vi "Pump Status Pump Module.vi"(8 "error in (no error)":errorcluster, 11 "?":T1={"State"=enum."Idle", "Start Time"=timestamp(0 s since 1904-01-01), "Configuration"={"Cycle Period"=0.0, "Manual Entry"=0.0, "Output Device"=enum."VICI M6", "Ismatech"={"VISA resource name"="", "Simulated?"=FALSE, "Pump Number"=1.0, "Reverse?"=FALSE}, "Ismatech 3 Channel Settings"={"VISA resource name"="", "Pump Number"=1, "Channel Number"=0, "Simulated?"=TRUE, "Reverse?"=FALSE}, "Masterflex"={"VISA resource name"="", "Simulated?"=FALSE, "Pump Number"=1.0, "Reverse?"=FALSE}, "VICI Settings"={"VISA resource name"="", "Pump ID"="", "Pump Head Vol"=0.0, "Reverse?"=FALSE, "Simulated?"=FALSE}, "Tacmina Settings"={"Analog DAQ Task"="", "Digital DAQ Task"=""}, "KNF SIMDOS Settings"={"VISA resource name"="", "Simulated?"=TRUE}, "ASIA Pump C"={"ASIA Pump #"=0, "channel"=0, "Simulated"=FALSE}, "FLOM Settings"={"VISA resource name"="", "Simulated?"=TRUE, "Pump Number"=0.0}, "SSI PR/LD Settings"={"VISA resource name"="", "Simulated?"=FALSE}, "SSI P40 Settings"={"VISA resource name"="", "Simulated?"=FALSE}, "Masterflex 75211 Settings"={"Analog DAQ Task"="", "Digital DAQ Task"=""}, "Pump Calibration File"=path "", "Calibration Slope"=0.0, "Calibration Y Intercept"=0.0, "Pump Cal Enum"=0, "Reset Totalizer"=FALSE}, "Current Time"=timestamp(0 s since 1904-01-01), "First Iteration"=FALSE, "Data"={"Pump Speed"=0.0, "Pump Pressure"=0.0, "Pump Flow"=0.0, "Totalized"=0.0}, "Process Name"="", "Pump On?"=enum."Off", "Output Error"=FALSE, "Log Started"=FALSE, "Overpressure Alarming"=FALSE} {"Configuration"."Ismatech 3 Channel Settings"."Channel Number" min=0 max=3; "Configuration"."Ismatech 3 Channel Settings"."Pump Number" min=1; "Configuration"."ASIA Pump C"."channel" min=0 max=1 step=1; "Configuration"."Masterflex"."Pump Number" min=1.0 max=20.0 step=1.0; "Configuration"."Ismatech"."Pump Number" min=1.0 max=20.0 step=1.0}) -> (0 "error out":errorcluster, 3 "State out":T1={"State"=enum."Idle", "Start Time"=timestamp(0 s since 1904-01-01), "Configuration"={"Cycle Period"=0.0, "Manual Entry"=0.0, "Output Device"=enum."Ismatec ISM 831C", "Ismatech"={"VISA resource name"="", "Simulated?"=FALSE, "Pump Number"=1.0, "Reverse?"=FALSE}, "Ismatech 3 Channel Settings"={"VISA resource name"="", "Pump Number"=1, "Channel Number"=0, "Simulated?"=TRUE, "Reverse?"=FALSE}, "Masterflex"={"VISA resource name"="", "Simulated?"=FALSE, "Pump Number"=1.0, "Reverse?"=FALSE}, "VICI Settings"={"VISA resource name"="", "Pump ID"="", "Pump Head Vol"=0.0, "Reverse?"=FALSE, "Simulated?"=FALSE}, "Tacmina Settings"={"Analog DAQ Task"="", "Digital DAQ Task"=""}, "KNF SIMDOS Settings"={"VISA resource name"="", "Simulated?"=TRUE}, "ASIA Pump C"={"ASIA Pump #"=0, "channel"=0, "Simulated"=FALSE}, "FLOM Settings"={"VISA resource name"="", "Simulated?"=TRUE, "Pump Number"=0.0}, "SSI PR/LD Settings"={"VISA resource name"="", "Simulated?"=FALSE}, "SSI P40 Settings"={"VISA resource name"="", "Simulated?"=FALSE}, "Masterflex 75211 Settings"={"Analog DAQ Task"="", "Digital DAQ Task"=""}, "Pump Calibration File"=path "", "Calibration Slope"=0.0, "Calibration Y Intercept"=0.0, "Pump Cal Enum"=0, "Reset Totalizer"=FALSE}, "Current Time"=timestamp(0 s since 1904-01-01), "First Iteration"=FALSE, "Data"={"Pump Speed"=0.0, "Pump Pressure"=0.0, "Pump Flow"=0.0, "Totalized"=0.0}, "Process Name"="", "Pump On?"=enum."Off", "Output Error"=FALSE, "Log Started"=FALSE, "Overpressure Alarming"=FALSE} {"Configuration"."Ismatech 3 Channel Settings"."Channel Number" min=0 max=3; "Configuration"."Ismatech 3 Channel Settings"."Pump Number" min=1; "Configuration"."ASIA Pump C"."channel" min=0 max=1 step=1; "Configuration"."Masterflex"."Pump Number" min=1.0 max=20.0 step=1.0; "Configuration"."Ismatech"."Pump Number" min=1.0 max=20.0 step=1.0})   [LabVIEW 2018, in "Pump Module.lvlib"]
uses:
  Pump Module.lvlib
  Measure Instrument/State Cluster.ctl
  Measure Instrument/State Enum.ctl
  Pump Module Settings Cluster.ctl
  Measure Instrument/PID 2 Output Enum.ctl
  Ismatec ISM 831C/Controls/Ismatech ISM831C Settings Cluster.ctl
  Ismatec 78001/Ismatec 4083.ctl
  Masterflex 7550-30/Controls/Settings Cluster.ctl
  VICI M50 Party Mode/Settings Cluster.ctl
  Tacmina QI/Tacmina QI DAQ Setting.ctl
  KNF Pump/Settings Cluster plus SIMDOS.ctl
  ASIA Pump/Pump Settings.ctl
  FLOM Pump/Settings Cluster.ctl
  SSI PR Class/SSI PR or LD Settings Cluster.ctl
  Masterflex 75211/Masterflex 75211 DAQ Setting.ctl
  Tag VIs/Tag FGV Operation Enum.ctl
  Ismatec ISM 831C/Ismatec ISM 831C.lvlib
  Masterflex 7550-30/Masterflex 7550-30.lvlib
  Shared Variables/Dynamic Shared Variables.lvlib
  Measure Instrument/Pump Module Engine.lvlib
  Tacmina QI/Tacmina QI.lvlib
  KNF Pump/KNF SIMDOS.lvlib
  VICI M50 Party Mode/VICI M6 M50 Party Mode.lvlib
  FLOM Pump/FLOM Pump.lvlib
  ASIA Pump.lvlib
  SSI PR Class/SSI PR or LD Pump.lvlib
  Masterflex 75211/Masterflex 75211.lvlib
  SSI PR Class/SSI P40 Pump.lvlib
  Ismatec 78001/Ismatec 4308.lvlib
panel:
  # "Output Instruments"
  # "Output Instruments"
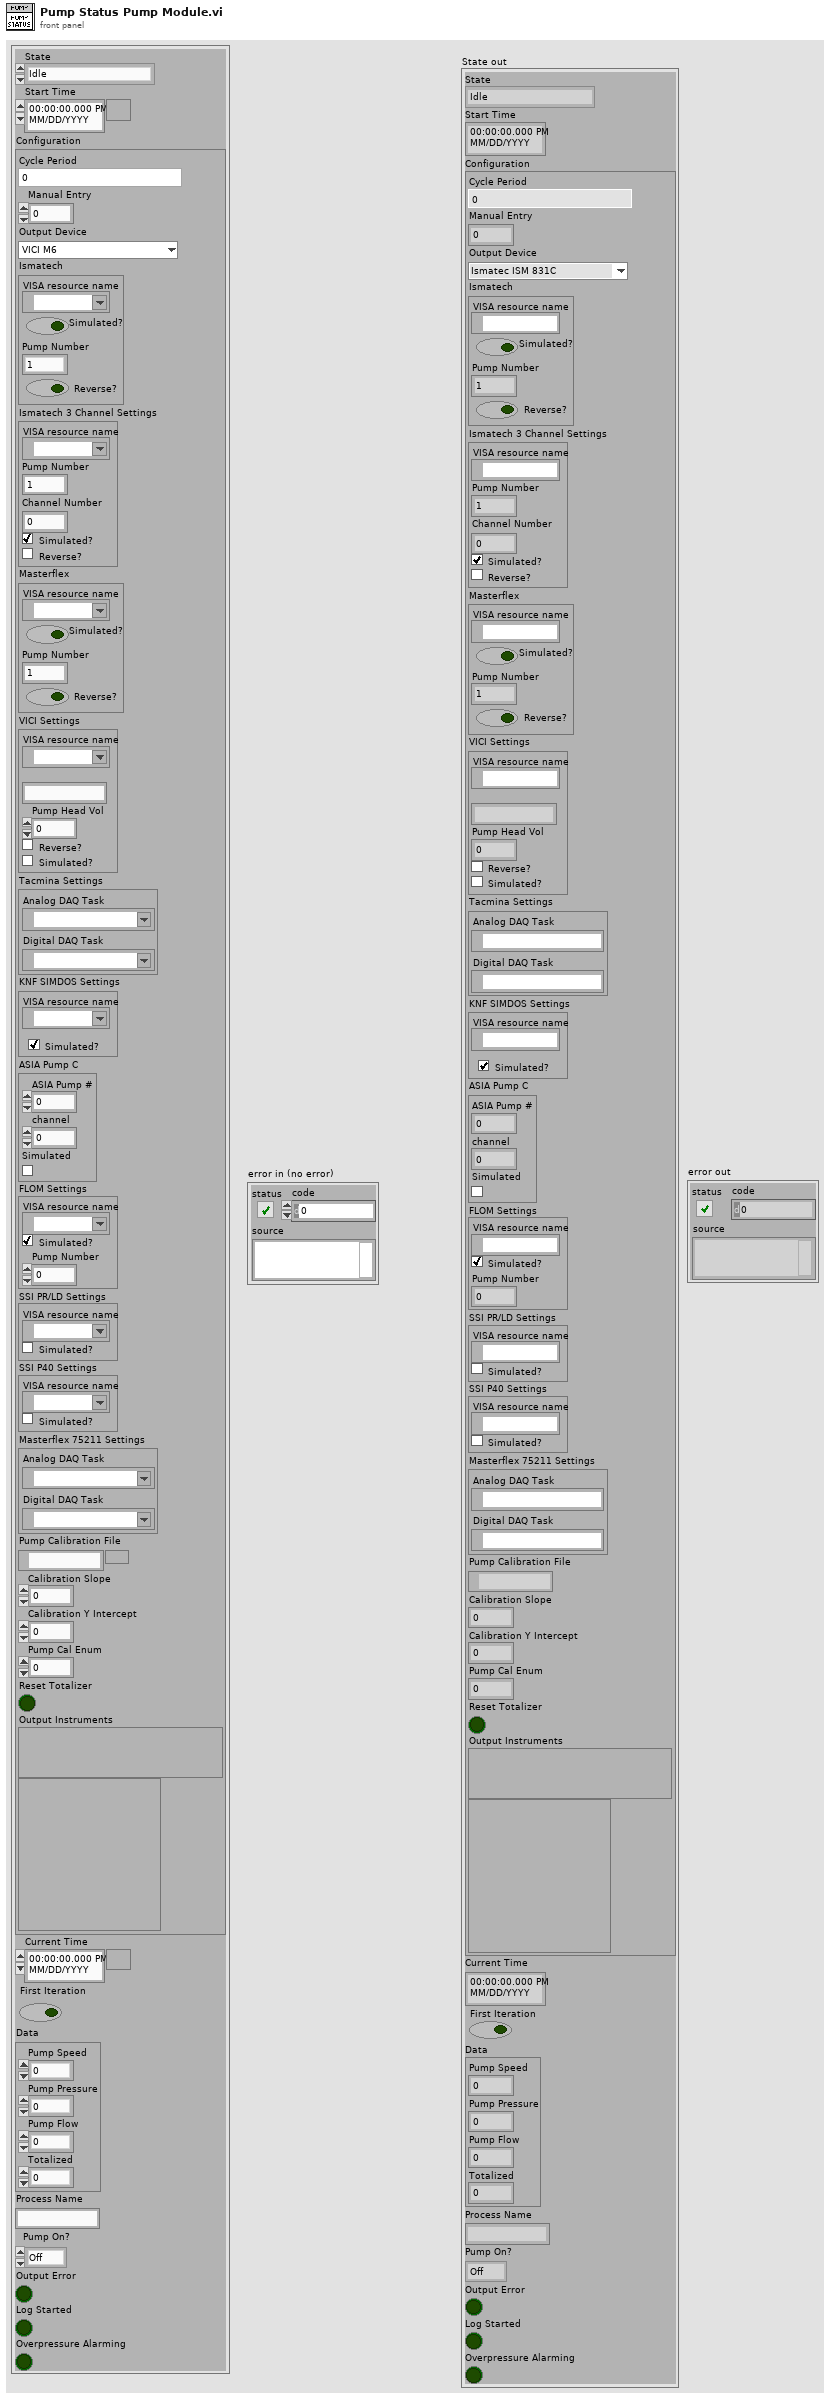
[diagram p1: front panel]
types:
  T1 = typedef "Pump Module.lvlib/Pump Module Engine.lvlib/State Cluster.ctl" = cluster{"State":T2, "Start Time":timestamp, "Configuration":T3, "Current Time":timestamp, "First Iteration":bool, "Data":cluster{"Pump Speed":dbl, "Pump Pressure":dbl, "Pump Flow":dbl, "Totalized":dbl}, "Process Name":string, "Pump On?":enum16{"Off", "On", "Not Initialized"}, "Output Error":bool, "Log Started":bool, "Overpressure Alarming":bool}
  T2 = typedef "Pump Module.lvlib/Pump Module Engine.lvlib/State Enum.ctl" = enum16{"Measuring", "Idle", "Paused"}
  T3 = typedef "Pump Module.lvlib/Pump Module Settings Cluster.ctl" = cluster{"Cycle Period":dbl, "Manual Entry":dbl, "Output Device":T4, "Ismatech":T5, "Ismatech 3 Channel Settings":T6, "Masterflex":T7, "VICI Settings":T8, "Tacmina Settings":T9, "KNF SIMDOS Settings":T10, "ASIA Pump C":T11, "FLOM Settings":T12, "SSI PR/LD Settings":T13, "SSI P40 Settings":T13, "Masterflex 75211 Settings":T14, "Pump Calibration File":path, "Calibration Slope":dbl, "Calibration Y Intercept":dbl, "Pump Cal Enum":u16, "Reset Totalizer":bool}
  T4 = typedef "PID 2 Output Enum.ctl" = enum16{"Default", "Ismatec ISM 4308", "Ismatec ISM 831C", "Masterflex 7550-30", "VICI M6", "VICI M50", "Tacmina QI", "KNF SIMDOS", "ASIA Type C", "FLOM UI-22-11", "SSI PR/LD", "SSI P40", "Masterflex 75211-70"}
  T5 = typedef "Ismatec ISM 831C.lvlib/Ismatech ISM831C Settings Cluster.ctl" = cluster{"VISA resource name":refnum<visa-resource-name>, "Simulated?":bool, "Pump Number":dbl, "Reverse?":bool}
  T6 = typedef "Ismatec 4308.lvlib/Ismatec 4083.ctl" = cluster{"VISA resource name":refnum<visa-resource-name>, "Pump Number":i16, "Channel Number":i16, "Simulated?":bool, "Reverse?":bool}
  T7 = typedef "Masterflex 7550-30.lvlib/Settings Cluster.ctl" = cluster{"VISA resource name":refnum<visa-resource-name>, "Simulated?":bool, "Pump Number":dbl, "Reverse?":bool}
  T8 = typedef "VICI M6 M50 Party Mode.lvlib/Settings Cluster.ctl" = cluster{"VISA resource name":refnum<visa-resource-name>, "Pump ID":string, "Pump Head Vol":dbl, "Reverse?":bool, "Simulated?":bool}
  T9 = typedef "Tacmina QI.lvlib/Tacmina QI DAQ Setting.ctl" = cluster{"Analog DAQ Task":refnum<k21>, "Digital DAQ Task":refnum<k21>}
  T10 = typedef "KNF SIMDOS.lvlib/Settings Cluster plus SIMDOS.ctl" = cluster{"VISA resource name":refnum<visa-resource-name>, "Simulated?":bool}
  T11 = typedef "ASIA Pump.lvlib/Pump Settings.ctl" = cluster{"ASIA Pump #":i32, "channel":i32, "Simulated":bool}
  T12 = typedef "FLOM Pump.lvlib/Settings Cluster.ctl" = cluster{"VISA resource name":refnum<visa-resource-name>, "Simulated?":bool, "Pump Number":dbl}
  T13 = typedef "SSI PR or LD Pump.lvlib/SSI PR or LD Settings Cluster.ctl" = cluster{"VISA resource name":refnum<visa-resource-name>, "Simulated?":bool}
  T14 = typedef "Masterflex 75211.lvlib/Masterflex 75211 DAQ Setting.ctl" = cluster{"Analog DAQ Task":refnum<k21>, "Digital DAQ Task":refnum<k21>}
  T15 = typedef "Tag FGV Operation Enum.ctl" = enum16{"Init", "Set Notification Queue", "Create Tag", "Commit", "Write Tag (Numeric)", "Write Tag (Boolean)", "Read All Tags", "Read One Tag", "Delete Tag Category", "Set Alarm Parameters (Numeric)", "Set Alarm Parameters (Boolean)", "Enable All Alarms", "Disable All Alarms", "Delete All Tags", "Read Alarms", "Ack Alarm", "Read Alarm Parameters (Numeric)", "Read Alarm Parameters (Boolean)"}
  T16 = typedef "Pump Module.lvlib/Pump Module Tag Names Cluster.ctl" = cluster{"Pump Speed":string, "Totalized g Tag":string, "Pump Flow":string, "Pump Pressure":string, "Output Device Tag":string, "Overpressure Tag":string, "Identifier Tag":string}
  T17 = cluster{"alarm URL":string, "set time":timestamp, "set user":string, "ack time":timestamp, "ack user":string, "clear time":timestamp, "clear user":string, "setpoint":dbl, "value":dbl, "priority":u32, "alarm area":string, "alarm description":string, "ack comment":string, "event?":bool, "Refnum":u64}[]
  T18 = typedef "Dynamic Shared Variables.lvlib/Alarm Cluster (UI).ctl" = cluster{"Color Box":u32, "Name":string, "Ack":bool}
  T19 = typedef "SSI P40 Pump.lvlib/SSI P40 Settings Cluster.ctl" = cluster{"VISA resource name":refnum<visa-resource-name>, "Simulated?":bool}
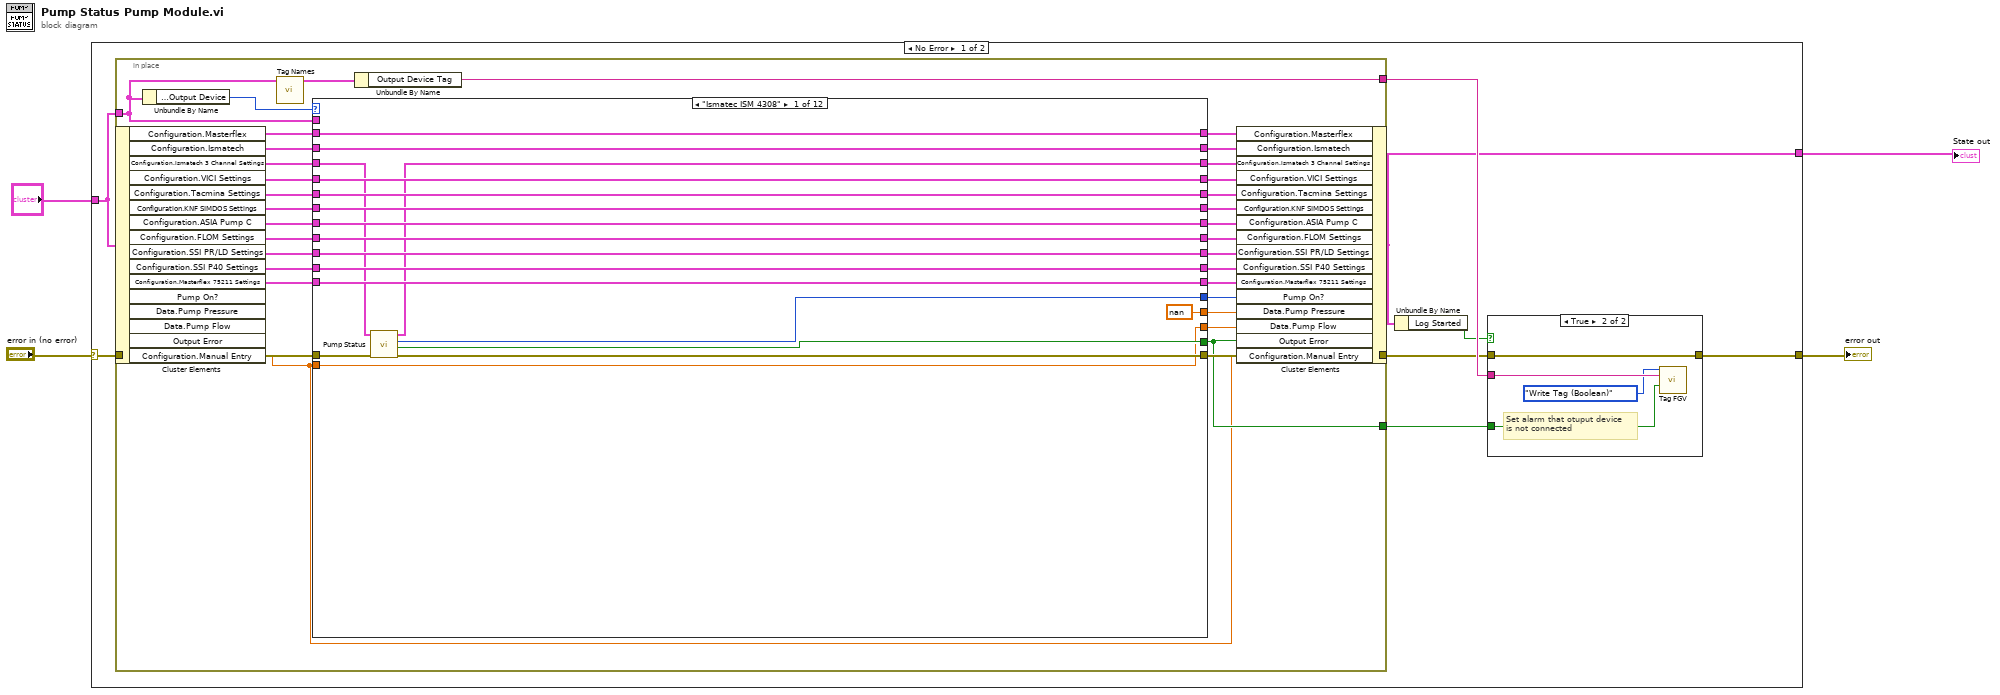
[diagram p0: block diagram]
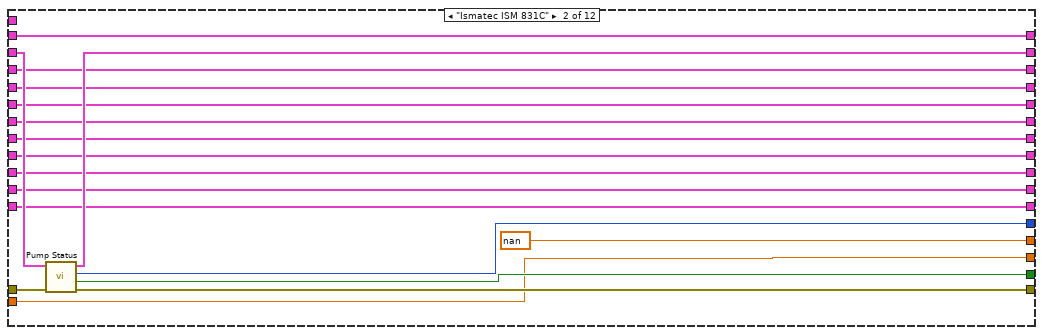
[diagram p2: hidden frame]
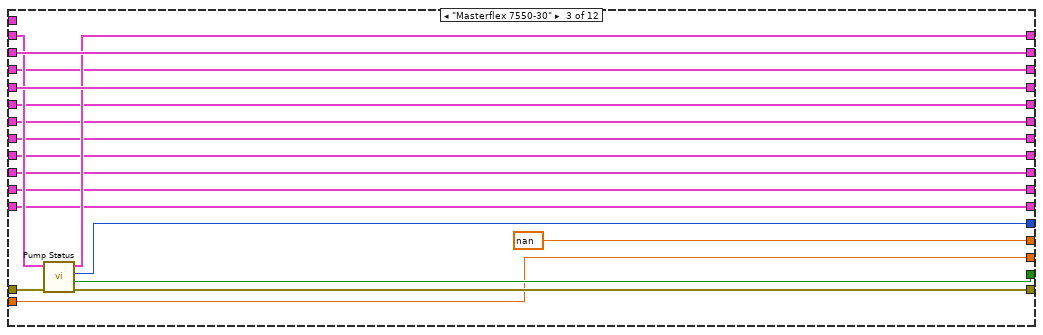
[diagram p3: hidden frame]
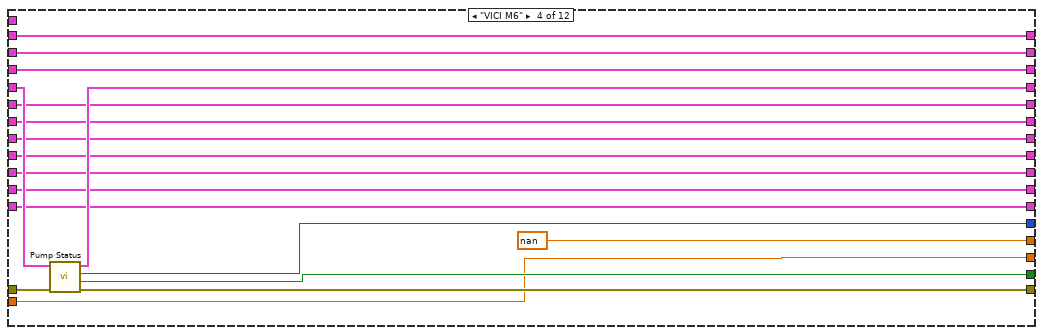
[diagram p4: hidden frame]
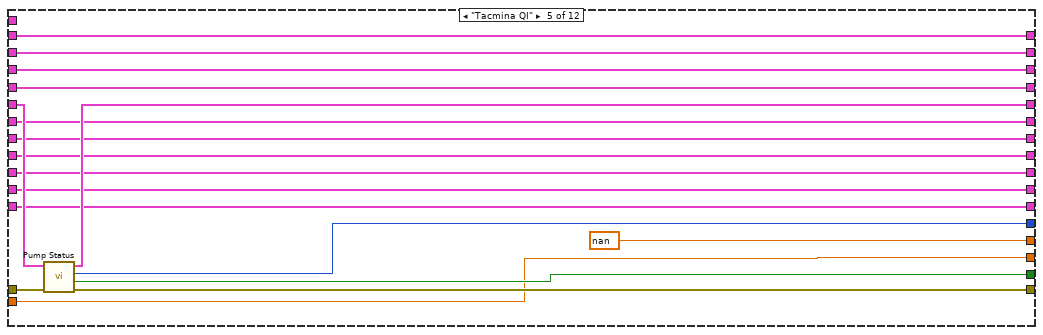
[diagram p5: hidden frame]
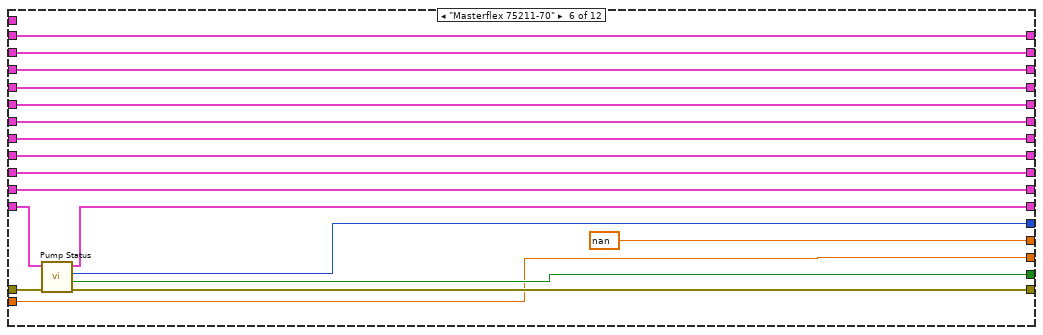
[diagram p6: hidden frame]
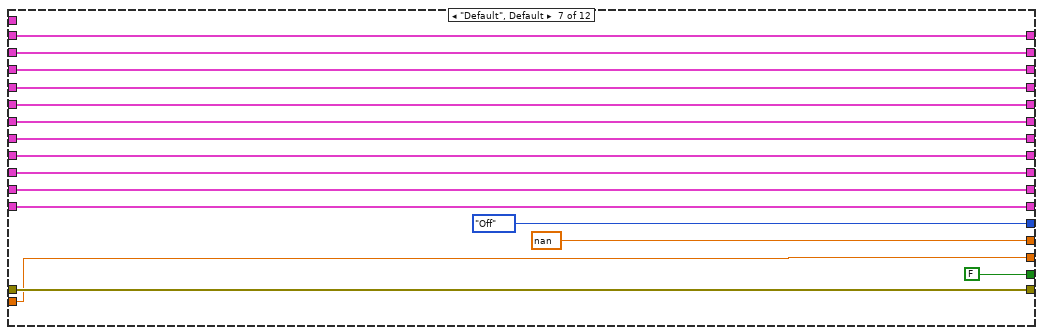
[diagram p7: hidden frame]
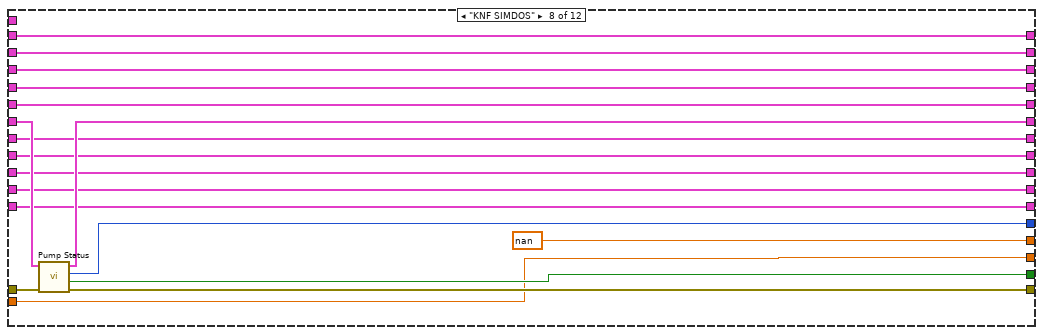
[diagram p8: hidden frame]
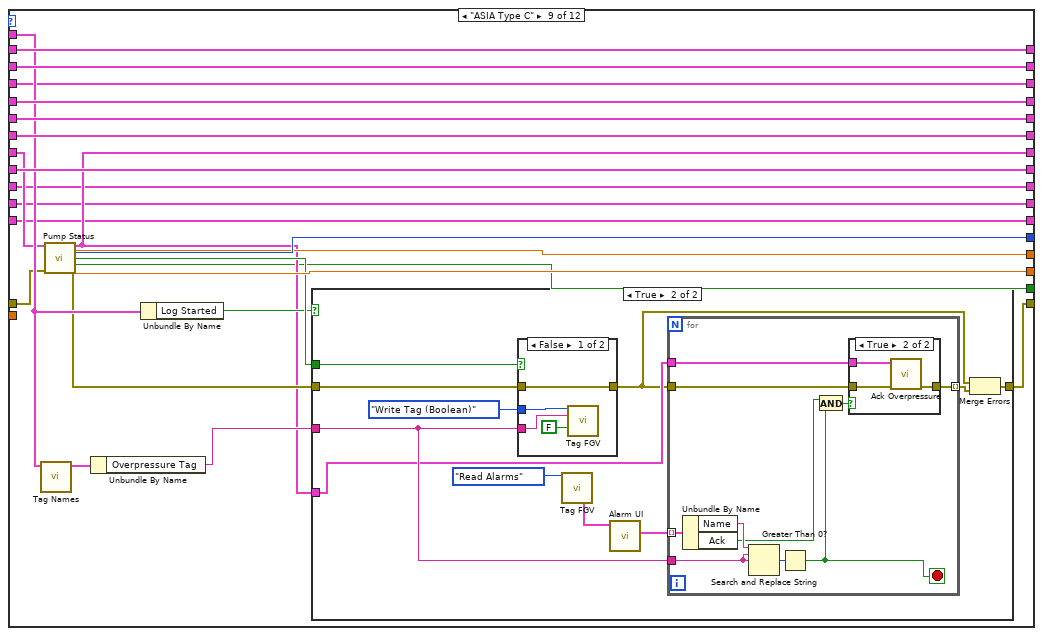
[diagram p9: hidden frame]
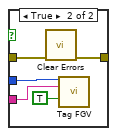
[diagram p12: hidden frame]
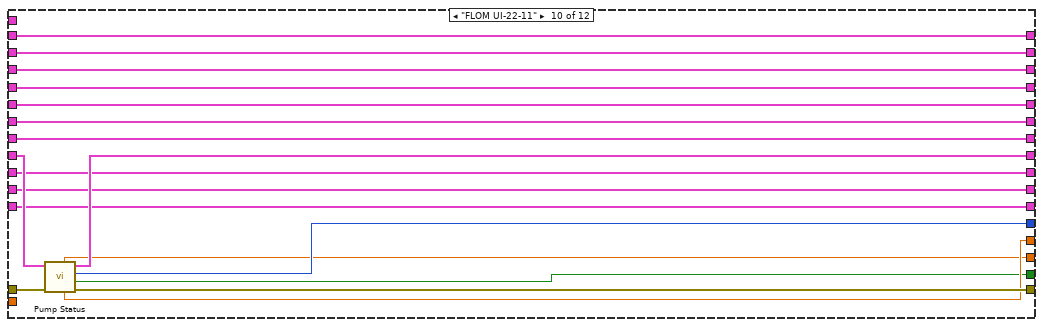
[diagram p13: hidden frame]
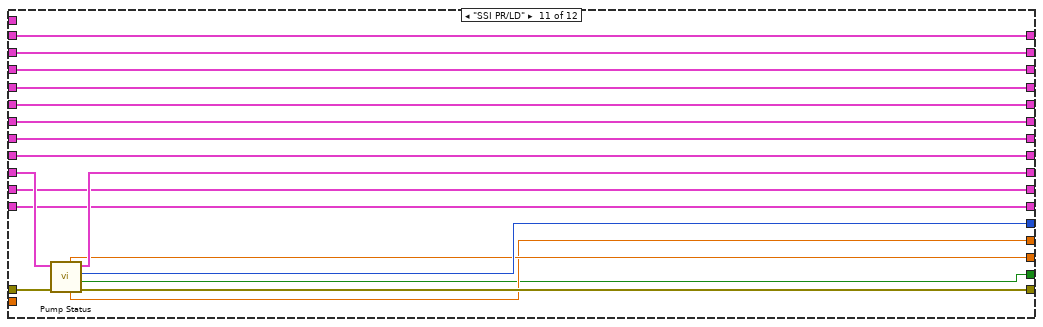
[diagram p14: hidden frame]
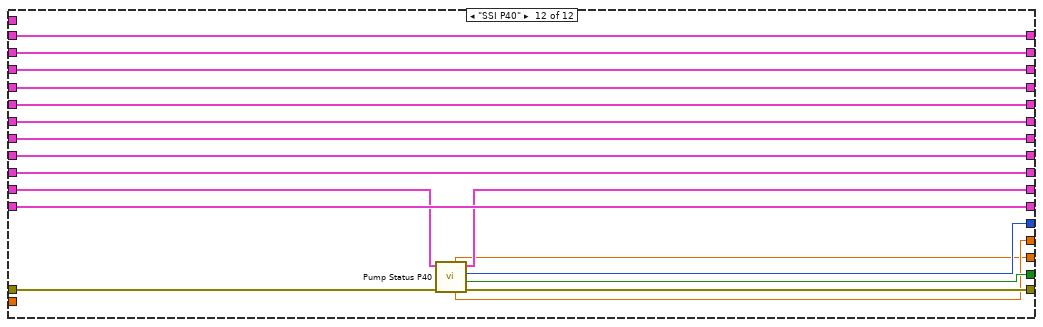
[diagram p15: hidden frame]
diagram:
  n1 = case shown="No Error" "error in (no error)" {
    selector: "error in (no error)" -> [w12 w307]
    tunnel: [w9 w307] -> w3
    tunnel: "?" -> [w6 w306]
    tunnel: [w5 w306] -> w1
    frame No Error {
      n2 = in-place {
        in-place-border: w12 -> [w45]
        in-place-border: [w44] -> w11
        in-place-border: [w43] -> w10
        in-place-border: w6 -> [w40]
        in-place-border: [w31] -> w7
        n3 = in-place-cluster #1(w6) -> ("Configuration.Masterflex"=w39:T7, "Configuration.Ismatech"=w38:T5, "Configuration.Ismatech 3 Channel Settings"=w16:T6, "Configuration.VICI Settings"=w37:T8, "Configuration.Tacmina Settings"=w36:T9, "Configuration.KNF SIMDOS Settings"=w35:T10, "Configuration.ASIA Pump C"=w34:T11, "Configuration.FLOM Settings"=w33:T12, "Configuration.SSI PR/LD Settings"=w32:T13, "Configuration.SSI P40 Settings"=w17:T13, "Configuration.Masterflex 75211 Settings"=w20:T14, "Configuration.Manual Entry"=w13:dbl)  [unwired: 4 out]
        n4 = Unbundle By Name(w40) -> ("Configuration.Output Device"=w41:T4)
        n5 = call "Tag Names.vi"("State In"=w40) -> ("Pump Module Tag Names"=w42:T16)  [unwired: 8 in, 2 out]
        n6 = case "Selected Device" shown="\"Ismatec ISM 4308\"" w41 {
          tunnel: w39 -> [w63 w81 w94 w116 w135 w153 w169 w187 w211 w264 w282 w292]
          tunnel: [w63 w81 w95 w116 w135 w153 w169 w187 w211 w264 w282 w292] -> w30
          tunnel: w38 -> [w62 w78 w99 w117 w134 w152 w168 w186 w210 w263 w281 w300]
          tunnel: [w50 w79 w96 w112 w130 w142 w166 w182 w194 w257 w272 w286] -> w43
          tunnel: w45 -> [w53 w80 w97 w113 w131 w145 w166 w183 w203 w258 w276 w291]
          tunnel: [w62 w77 w99 w117 w134 w152 w168 w186 w210 w263 w281 w300] -> w29
          tunnel: w37 -> [w61 w75 w98 w114 w133 w151 w167 w185 w209 w262 w280 w299]
          tunnel: [w61 w75 w98 w115 w133 w151 w167 w185 w209 w262 w280 w299] -> w28
          tunnel: w36 -> [w60 w76 w93 w111 w132 w141 w165 w184 w208 w261 w279 w298]
          tunnel: [w60 w76 w93 w111 w129 w141 w165 w184 w208 w261 w279 w298] -> w27
          tunnel: [w59 w74 w92 w110 w128 w150 w164 w181 w207 w260 w278 w297] -> w26
          tunnel: w35 -> [w59 w74 w92 w110 w128 w150 w164 w180 w207 w260 w278 w297]
          tunnel: [w48 w73 w90 w109 w127 w144 enum16{"Off", "On", "Not Initialized"}."Off" ("Pump On?") w179 w201 w254 w271 w288] -> w22
          tunnel: [w58 w72 w91 w108 w126 w149 w162 w178 w193 w259 w277 w296] -> w25
          tunnel: w34 -> [w58 w72 w91 w108 w126 w149 w162 w178 w202 w259 w277 w296]
          tunnel: [w57 w71 w89 w107 w125 w148 w161 w177 w206 w256 w275 w295] -> w24
          tunnel: w33 -> [w57 w71 w89 w107 w125 w148 w161 w177 w206 w255 w275 w295]
          tunnel: [w46 w64 w82 w100 w118 w136 w154 w170 w198 w252 w270 w284] -> w14
          tunnel: [nan ("Pressure") nan ("Pressure") nan ("Pressure") nan ("Pressure") nan ("Pressure") nan ("Pressure") nan ("Pressure") nan ("Pressure") w199 w253 w269 w285] -> w21
          tunnel: w40 -> [_ _ _ _ _ _ _ _ w204 _ _ _]
          tunnel: w32 -> [w56 w69 w87 w105 w123 w146 w159 w175 w192 w251 w274 w294]
          tunnel: [w56 w69 w87 w105 w123 w146 w159 w175 w192 w251 w273 w294] -> w23
          tunnel: [w49 w68 w86 w104 w122 w143 FALSE ("Connection Error") w174 w191 w250 w268 w287] -> w31
          tunnel: w20 -> [w55 w67 w85 w103 w121 w140 w157 w173 w190 w249 w267 w293]
          tunnel: [w55 w67 w85 w103 w121 w139 w157 w173 w190 w249 w267 w293] -> w19
          tunnel: [w54 w66 w84 w102 w120 w138 w156 w172 w189 w248 w266 w289] -> w18
          tunnel: w17 -> [w54 w66 w84 w102 w120 w138 w156 w172 w189 w248 w266 w290]
          tunnel: w16 -> [w52 w65 w83 w101 w119 w137 w155 w171 w188 w247 w265 w283]
          tunnel: [w51 w65 w83 w101 w119 w137 w155 w171 w188 w247 w265 w283] -> w15
          tunnel: w13 -> [w46 w64 w82 w100 w118 w136 w154 w170 _ _ _ _]
          frame "Ismatec ISM 4308" {
            n7 = call "Pump Status.vi"("error in (no error)"=w53, "Ismatech 3 Channel Settings In"=w52) -> ("error out"=w50:errorcluster, "Connection Error"=w49:bool, "Pump On?"=w48:enum16{"Off", "On", "Not Initialized"}, "Ismatech 3 Channel Settings Out"=w51:T6)  [unwired: 5 in, 1 out]
          }
          frame "Ismatec ISM 831C" {
            n8 = call "Pump Status.vi"("error in (no error)"=w80, "Ismatech Settings In"=w78) -> ("error out"=w79:errorcluster, "Connection Error"=w68:bool, "Pump On?"=w73:enum16{"Off", "On", "Not Initialized"}, "Ismatech Settings Out"=w77:T5)  [unwired: 6 in]
          }
          frame "Masterflex 7550-30" {
            n9 = call "Pump Status.vi"("error in (no error)"=w97, "Masterflex Settings in"=w94) -> ("error out"=w96:errorcluster, "Connection Error"=w86:bool, "Pump On?"=w90:enum16{"Off", "On", "Not Initialized"}, "Masterflex Settings out"=w95:T7)  [unwired: 6 in]
          }
          frame "VICI M6" {
            n10 = call "Pump Status.vi"("error in (no error)"=w113, "VICI Settings In"=w114) -> ("error out"=w112:errorcluster, "Connection Error"=w104:bool, "Pump On?"=w109:enum16{"Off", "On", "Not Initialized"}, "VICI Settings Out"=w115:T8)  [unwired: 6 in]
          }
          frame "Tacmina QI" {
            n11 = call "Pump Status.vi"("error in"=w131, "Tacmina Settings in"=w132) -> ("error out"=w130:errorcluster, "Connection Error"=w122:bool, "Pump On?"=w127:enum16{"Off", "On", "Not Initialized"}, "Tacmina Settings out"=w129:T9)  [unwired: 6 in]
          }
          frame "Masterflex 75211-70" {
            n12 = call "Pump Status.vi"("error in"=w145, "Masterflex 75211 Settings"=w140) -> ("error out"=w142:errorcluster, "Connection Error"=w143:bool, "Pump On?"=w144:enum16{"Off", "On", "Not Initialized"}, "Masterflex 75211 Settings"=w139:T14)  [unwired: 6 in]
          }
          frame "Default", Default {
          }
          frame "KNF SIMDOS" {
            n13 = call "Pump Status.vi"("error in (no error)"=w183, "KNF Settings In"=w180) -> ("error out"=w182:errorcluster, "Connection Error"=w174:bool, "Pump On?"=w179:enum16{"Off", "On", "Not Initialized"}, "KNF Settings Out"=w181:T10)  [unwired: 6 in]
          }
          frame "ASIA Type C" {
            n14 = call "Tag Names.vi"("State In"=w204) -> ("Pump Module Tag Names"=w205:T16)  [unwired: 8 in, 2 out]
            n15 = call "Pump Status.vi"("ASIA Pump C Settings in"=w202, "error in (no error)"=w203) -> ("pressure"=w199:dbl, "ASIA Pump C Settings out"=w193:T11, "Pump On?"=w201:enum16{"Off", "On", "Not Initialized"}, "Overpressure"=w197:bool, "Connection Error"=w191:bool, "pumpRate"=w198:dbl, "error out"=w200:errorcluster)  [unwired: 5 in, 2 out]
            n16 = Unbundle By Name(w205) -> ("Overpressure Tag"=w195:string)
            n17 = Unbundle By Name(w204) -> ("Log Started"=w196:bool)
            n18 = case shown="True" w196 {
              tunnel: w195 -> [_ w217]
              tunnel: w200 -> [w212 w223]
              tunnel: w197 -> [_ w222]
              tunnel: [w212 w214] -> w194
              tunnel: w193 -> [_ w216]
              frame False {
              }
              frame True {
                n19 = case shown="False" w222 {
                  tunnel: Tag_FGV_Operation_Enum."Write Tag (Boolean)" ("Operation") -> [w241 w246]
                  tunnel: w217 -> [w240 w245]
                  tunnel: [w239 w243] -> w213
                  tunnel: w223 -> [w239 w244]
                  frame False {
                    n20 = call "Tag FGV.vi"("Operation"=w241, "Tag Name"=w240, "Data"=FALSE) -> ()  [unwired: 5 in, 8 out]
                  }
                  frame True {
                    n21 = call <vilib>:"Clear Errors.vi"("error in (no error)"=w244) -> ("error out"=w243:errorcluster)  [unwired: 5 in, 1 out]
                    n22 = call "Tag FGV.vi"("Operation"=w246, "Tag Name"=w245, "Data"=TRUE) -> ()  [unwired: 5 in, 8 out]
                  }
                }
                n23 = call "Tag FGV.vi"("Operation"=Tag_FGV_Operation_Enum."Read Alarms") -> ("alarms"=w219:T17)  [unwired: 7 in, 7 out]
                n24 = call "Alarm UI.vi"("alarms"=w219) -> ("UI Alarms"=w218:T18[])  [unwired: 9 in, 1 out]
                n25 = for {
                  tunnel: w218 -> [w233] mode=indexing
                  tunnel: w217 -> [w230]
                  tunnel: w216 -> [w229]
                  tunnel: [w228] -> w215 mode=indexing
                  tunnel: w213 -> [w227]
                  stop <- w225 stop-if-true
                  n26 = Unbundle By Name(w233) -> ("Name"=w232:string, "Ack"=w224:bool)
                  n27 = Search and Replace String(input string=w232, search string=w230, replace string=w230) -> (number of replacements=w231:i32)  [unwired: 5 in, 3 out]
                  n28 = Greater Than 0?(x=w231) -> (x > 0?=w225:bool)
                  n29 = And(x=w224, y=w225) -> (x .and. y?=w226:bool)
                  n30 = case shown="True" w226 {
                    tunnel: w229 -> [_ w237]
                    tunnel: [w234 w236] -> w228
                    tunnel: w227 -> [w234 w235]
                    frame False {
                    }
                    frame True {
                      n31 = call "Ack Overpressure.vi"("error in (no error)"=w235, "ASIA Pump C Settings in"=w237) -> ("error out"=w236:errorcluster)  [unwired: 9 in]
                    }
                  }
                }
                n32 = Merge Errors(w213, w215) -> (w214:errorcluster)
              }
            }
          }
          frame "FLOM UI-22-11" {
            n33 = call "Pump Status.vi"("error in (no error)"=w258, "FLOM Settings In"=w255) -> ("error out"=w257:errorcluster, "Connection Error"=w250:bool, "Pump On?"=w254:enum16{"Off", "On", "Not Initialized"}, "FLOM Settings Out"=w256:T12, "Pressure"=w253:dbl, "Flow Rate"=w252:dbl)  [unwired: 4 in]
          }
          frame "SSI PR/LD" {
            n34 = call "Pump Status.vi"("error in (no error)"=w276, "SSI PR Settings"=w274) -> ("error out"=w272:errorcluster, "Connection Error"=w268:bool, "Pump On?"=w271:enum16{"Off", "On", "Not Initialized"}, "SSI PR Settings"=w273:T13, "Pressure"=w269:dbl, "Flow"=w270:dbl)  [unwired: 4 in]
          }
          frame "SSI P40" {
            n35 = call "Pump Status P40.vi"("error in (no error)"=w291, "SSI P40 Settings In"=w290) -> ("error out"=w286:errorcluster, "Connection Error"=w287:bool, "Pump On?"=w288:enum16{"Off", "On", "Not Initialized"}, "SSI P40 Settings Out"=w289:T19, "Pressure"=w285:dbl, "Flow"=w284:dbl)  [unwired: 4 in]
          }
        }
        n36 = Unbundle By Name(w42) -> ("Output Device Tag"=w44:string)
        n37 = in-place-cluster #1("Configuration.Masterflex"=w30, "Configuration.Ismatech"=w29, "Configuration.Ismatech 3 Channel Settings"=w15, "Configuration.VICI Settings"=w28, "Configuration.Tacmina Settings"=w27, "Configuration.KNF SIMDOS Settings"=w26, "Configuration.ASIA Pump C"=w25, "Configuration.FLOM Settings"=w24, "Configuration.SSI PR/LD Settings"=w23, "Configuration.SSI P40 Settings"=w18, "Configuration.Masterflex 75211 Settings"=w19, "Pump On?"=w22, "Data.Pump Pressure"=w21, "Data.Pump Flow"=w14, "Output Error"=w31, "Configuration.Manual Entry"=w13) -> (w5:T1)
      }
      n38 = Unbundle By Name(w5) -> ("Log Started"=w8:bool)
      n39 = case shown="True" w8 {
        tunnel: w11 -> [_ w305]
        tunnel: w10 -> [w301 w304]
        tunnel: [w301 w304] -> w9
        tunnel: w7 -> [_ w302]
        frame False {
        }
        frame True {
          # "Set alarm that otuput device\nis not connected"
          n40 = call "Tag FGV.vi"("Operation"=Tag_FGV_Operation_Enum."Write Tag (Boolean)", "Tag Name"=w305, "Data"=w302) -> ()  [unwired: 5 in, 8 out]
        }
      }
    }
    frame Error {
    }
  }
  "error out" <- w3
  "State out" <- w1
